vi "20 Chapter-Power Spectrum Measurement.vi"() -> ()   [LabVIEW 2014]
uses:
  <vilib>/Analysis/4window.llb/windowTd.ctl
  <vilib>/measure/maspectr.llb/FFT Power Spectrum for 1 Chan.vi
  <vilib>/measure/maspectr.llb/FFT Power Spectral Density for 1 Chan.vi
  <vilib>/measure/NI_MABase.lvlib
  <vilib>/measure/NI_MAPro.lvlib
  <vilib>/Analysis/NI_AALPro.lvlib
panel:
  in  "选项卡控件2":enum32{"FFT功率谱密度", "FFT功率谱"}(tab)
  out "FFT功率谱密度":cluster{"f0":dbl, "df":dbl, "magnitude":dbl[]}(graph)
  out "FFT功率谱":cluster{"f0":dbl, "df":dbl, "magnitude":dbl[]}(graph)
  in  "选项卡控件":enum32{"时间信号", "FFT功率谱密度/FFT功率谱"}(tab)
  in  "频率":dbl(knob)=3000.0 caption="频率(Hz)" min=0.0 max=10000.0 scale=0.0..10000.0
  in  "幅值":dbl=1.0 format="%0.2p"
  in  "重置信号":bool
  in  "波形信息":cluster{"Fs":dbl, "#s":dbl}={"Fs"=25600.0, "#s"=1024.0} caption="采样信息" {"Fs" format="%#.1f"}
  in  "标准偏差":dbl=1.0 format="%.3f"
  in  "窗":T1=1 items=["矩形"=0, "Hanning"=1, "Hamming"=2, "Blackman-Harris"=3, "Exact Blackman"=4, "Blackman"=5, "Flat Top"=6, "4阶Blackman-Harris "=7, "7阶Blackman-Harris"=8, "Low Sidelobe"=9, "Blackman Nuttall"=11, "三角"=30, "Bartlett-Hanning"=31, "Bohman"=32, "Parzen"=33, "Welch"=34, "Kaiser"=60, "Dolph-Chebyshev"=61, "高斯"=62]
  in  "平均参数":T2={"averaging mode"=enum."No averaging", "weighting mode"=enum."Exponential", "number of averages"=10} {"number of averages" min=1}
  out "完成平均":bool
  out "已完成平均":dbl caption="已完成平均数"
  in  "restart averaging (F)":bool caption="重新开始平均(F)"
  in  "dB On (F)":bool caption="显示为dB(F)"
  out "输入信号":waveform(dbl)(graph)
  in  "停止":bool
  # "信号的频谱分析"
  # "Input"
  # "Output"
  # "OFF"
  # "ON"
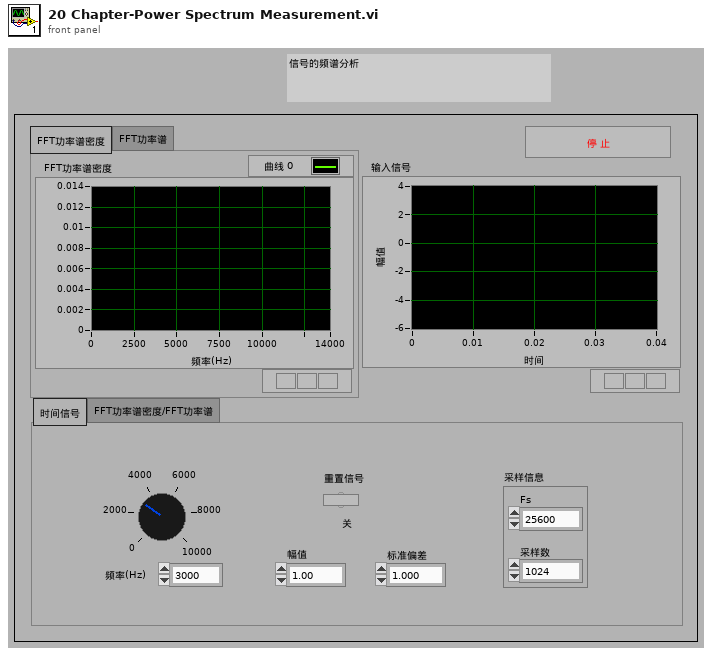
[diagram p1: front panel]
types:
  T1 = typedef "NI_AALPro.lvlib/windowTd.ctl" = u32
  T2 = cluster{"averaging mode":enum16{"No averaging", "Vector averaging", "RMS averaging", "Peak hold"}, "weighting mode":enum16{"Linear", "Exponential"}, "number of averages":u32}
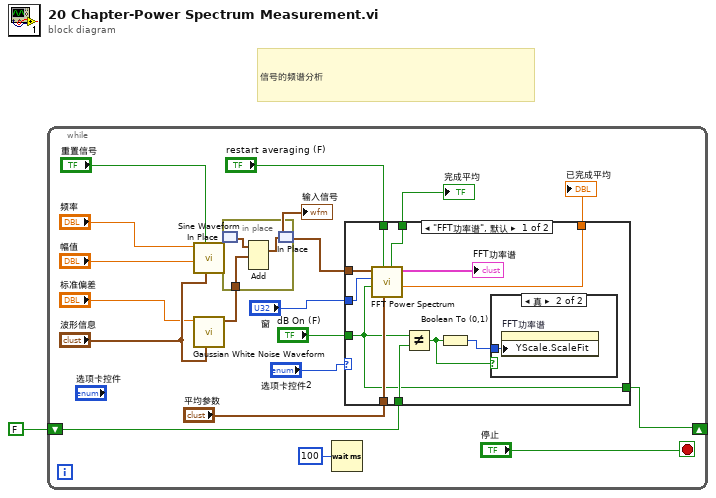
[diagram p0: block diagram]
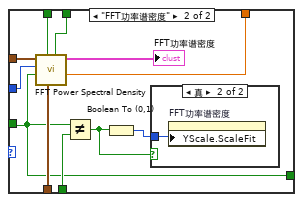
[diagram p3: hidden frame]
diagram:
  # "信号的频谱分析"
  n1 = while {
    shift-right: [w6] -> _
    shift-left: FALSE -> [w7]
    stop <- "停止" stop-if-true
    n2 = call <vilib>:"Sine Waveform.vi"("sampling info"="波形信息", "reset signal"="重置信号", "amplitude"="幅值", "frequency"="频率") -> ("signal out"=w20:waveform(dbl))  [unwired: 6 in, 1 out]
    n3 = call <vilib>:"Gaussian White Noise Waveform.vi"("sampling info"="波形信息", "standard deviation"="标准偏差") -> ("signal out"=w19:waveform(dbl))  [unwired: 8 in, 1 out]
    n4 = in-place {
      in-place-border: w19 -> [w22]
      n5 = in-place-match #1(w20) -> (w23:waveform(dbl))
      n6 = Add(1:w22, 2:w23) -> (0:w21:waveform(dbl))  [unwired: 1 in, 1 out]
      n7 = in-place-match #1(w21) -> (w2:waveform(dbl))
    }
    "输入信号" <- w2
    n8 = Wait (ms)(milliseconds to wait=u32 100 ("等待时间（毫秒）")) -> ()  [unwired: 1 out]
    n9 = case shown="\"FFT功率谱\", 默认" "选项卡控件2" {
      tunnel: w2 -> [w34 w41]
      tunnel: "窗" -> [w33 w39]
      tunnel: "dB On (F)" -> [w26 w38]
      tunnel: "平均参数" -> [w32 w40]
      tunnel: "restart averaging (F)" -> [w31 w44]
      tunnel: [w30 w43] -> w4
      tunnel: w7 -> [w29 w42]
      tunnel: [w26 w38] -> w6
      tunnel: [w24 w37] -> w5
      frame "FFT功率谱", Default {
        n10 = call-poly <vilib>:"FFT Power Spectrum.vi"("averaging parameters"=w32, "restart averaging (F)"=w31, "dB On (F)"=w26, "window"=w33, "time signal"=w34) -> ("averages completed"=w30:dbl, "power spectrum"=→"FFT功率谱":cluster{"f0":dbl, "df":dbl, "magnitude":dbl[]}, "averaging done"=w24:bool)  [unwired: 3 in, 1 out]
        n11 = Not Equal?(x=w26, y=w29) -> (x != y?=w27:bool)
        n12 = Boolean To (0,1)(Boolean=w27) -> (0, 1=w28:i16)
        n13 = case shown="真" w27 {
          tunnel: w28 -> [_ w35]
          frame False {
          }
          frame True {
            n14 = property on="FFT功率谱" class="WFGraph (严格)"("YScale.ScaleFit"=w35) -> ()  [unwired: 2 in, 2 out]
          }
        }
      }
      frame "FFT功率谱密度" {
        n15 = call-poly <vilib>:"FFT Power Spectral Density.vi"("averaging parameters"=w40, "restart averaging (F)"=w44, "dB On (F)"=w38, "window"=w39, "time signal"=w41) -> ("averages completed"=w43:dbl, "power spectral density"=→"FFT功率谱密度":cluster{"f0":dbl, "df":dbl, "magnitude":dbl[]}, "averaging done"=w37:bool)  [unwired: 3 in, 1 out]
        n16 = Not Equal?(x=w38, y=w42) -> (x != y?=w45:bool)
        n17 = Boolean To (0,1)(Boolean=w45) -> (0, 1=w46:i16)
        n18 = case shown="真" w45 {
          tunnel: w46 -> [_ w47]
          frame False {
          }
          frame True {
            n19 = property on="FFT功率谱密度" class="WFGraph (严格)"("YScale.ScaleFit"=w47) -> ()  [unwired: 2 in, 2 out]
          }
        }
      }
    }
    "已完成平均" <- w4
    "完成平均" <- w5
  }
